vi "MFLI_Merge_Cluster.vi"(3 "MFL_Monitor Control":T1 {"Osc 3 Freq" min=0.0 max=510000.0 format="%#_11g"; "Osc 2 Freq" min=0.0 max=510000.0 format="%#_11g"; "Osc 1 Freq" min=0.0 max=510000.0 format="%#_11g"; "Osc 0 Freq" min=0.0 max=510000.0 format="%#_11g"}, 5 "MFL_Monitor Status":T2 {"Demod Sample out 3"."Aux In 1 (V)" format="%#_5p"; "Demod Sample out 3"."Aux In 0 (V)" format="%#_5p"; "Demod Sample out 3"."X (Vrms)" format="%#_5p"; "Demod Sample out 3"."Y (Vrms)" format="%#_5p"; "Demod Sample out 3"."Osc Phase (rad)" format="%#.3g"; "Demod Sample out 2"."Aux In 1 (V)" format="%#_5p"; "Demod Sample out 2"."Aux In 0 (V)" format="%#_5p"; "Demod Sample out 2"."X (Vrms)" format="%#_5p"; "Demod Sample out 2"."Y (Vrms)" format="%#_5p"; "Demod Sample out 2"."Osc Phase (rad)" format="%#.3g"; "Demod Sample out 1"."Aux In 1 (V)" format="%#_5p"; "Demod Sample out 1"."Aux In 0 (V)" format="%#_5p"; "Demod Sample out 1"."X (Vrms)" format="%#_5p"; "Demod Sample out 1"."Y (Vrms)" format="%#_5p"; "Demod Sample out 1"."Osc Phase (rad)" format="%#.3g"; "Demod Sample out 0"."Aux In 1 (V)" format="%#_5p"; "Demod Sample out 0"."Aux In 0 (V)" format="%#_5p"; "Demod Sample out 0"."X (Vrms)" format="%#_5p"; "Demod Sample out 0"."Y (Vrms)" format="%#_5p"; "Demod Sample out 0"."Osc Phase (rad)" format="%#.3g"}) -> (1 "MFL_Monitor":T4 {"Osc 3 Freq" min=0.0 max=510000.0 format="%#_11g"; "Osc 2 Freq" min=0.0 max=510000.0 format="%#_11g"; "Osc 1 Freq" min=0.0 max=510000.0 format="%#_11g"; "Osc 0 Freq" min=0.0 max=510000.0 format="%#_11g"; "Demod Sample out 3"."Aux In 1 (V)" format="%#_5p"; "Demod Sample out 3"."Aux In 0 (V)" format="%#_5p"; "Demod Sample out 3"."X (Vrms)" format="%#_5p"; "Demod Sample out 3"."Y (Vrms)" format="%#_5p"; "Demod Sample out 3"."Osc Phase (rad)" format="%#.3g"; "Demod Sample out 2"."Aux In 1 (V)" format="%#_5p"; "Demod Sample out 2"."Aux In 0 (V)" format="%#_5p"; "Demod Sample out 2"."X (Vrms)" format="%#_5p"; "Demod Sample out 2"."Y (Vrms)" format="%#_5p"; "Demod Sample out 2"."Osc Phase (rad)" format="%#.3g"; "Demod Sample out 1"."Aux In 1 (V)" format="%#_5p"; "Demod Sample out 1"."Aux In 0 (V)" format="%#_5p"; "Demod Sample out 1"."X (Vrms)" format="%#_5p"; "Demod Sample out 1"."Y (Vrms)" format="%#_5p"; "Demod Sample out 1"."Osc Phase (rad)" format="%#.3g"; "Demod Sample out 0"."Aux In 1 (V)" format="%#_5p"; "Demod Sample out 0"."Aux In 0 (V)" format="%#_5p"; "Demod Sample out 0"."X (Vrms)" format="%#_5p"; "Demod Sample out 0"."Y (Vrms)" format="%#_5p"; "Demod Sample out 0"."Osc Phase (rad)" format="%#.3g"})   [LabVIEW 2019]
uses:
  zurich_lock_in/MFLIMonitor_Cluster.ctl
  Equipment/Zurich Instruments LabOne/Public/Data/ziTypeDemodSampleEx.ctl
  zurich_lock_in/MFLIMonitor_Status_Cluster.ctl
  zurich_lock_in/MFLIMonitor_Control_Cluster.ctl
  Equipment/Zurich Instruments LabOne/Zurich Instruments LabOne.lvlib
panel:
  # "Oscillators"
  # "Output Amplitudes"
  # "Frequency (Hz)"
  # "Ampl (Vpk)"
  # "0"
  # "0"
  # "1"
  # "1"
  # "2"
  # "2"
  # "3"
  # "3"
  # "Oscillators"
  # "Output Amplitudes"
  # "Frequency (Hz)"
  # "Ampl (Vpk)"
  # "0"
  # "0"
  # "1"
  # "1"
  # "2"
  # "2"
  # "3"
  # "3"
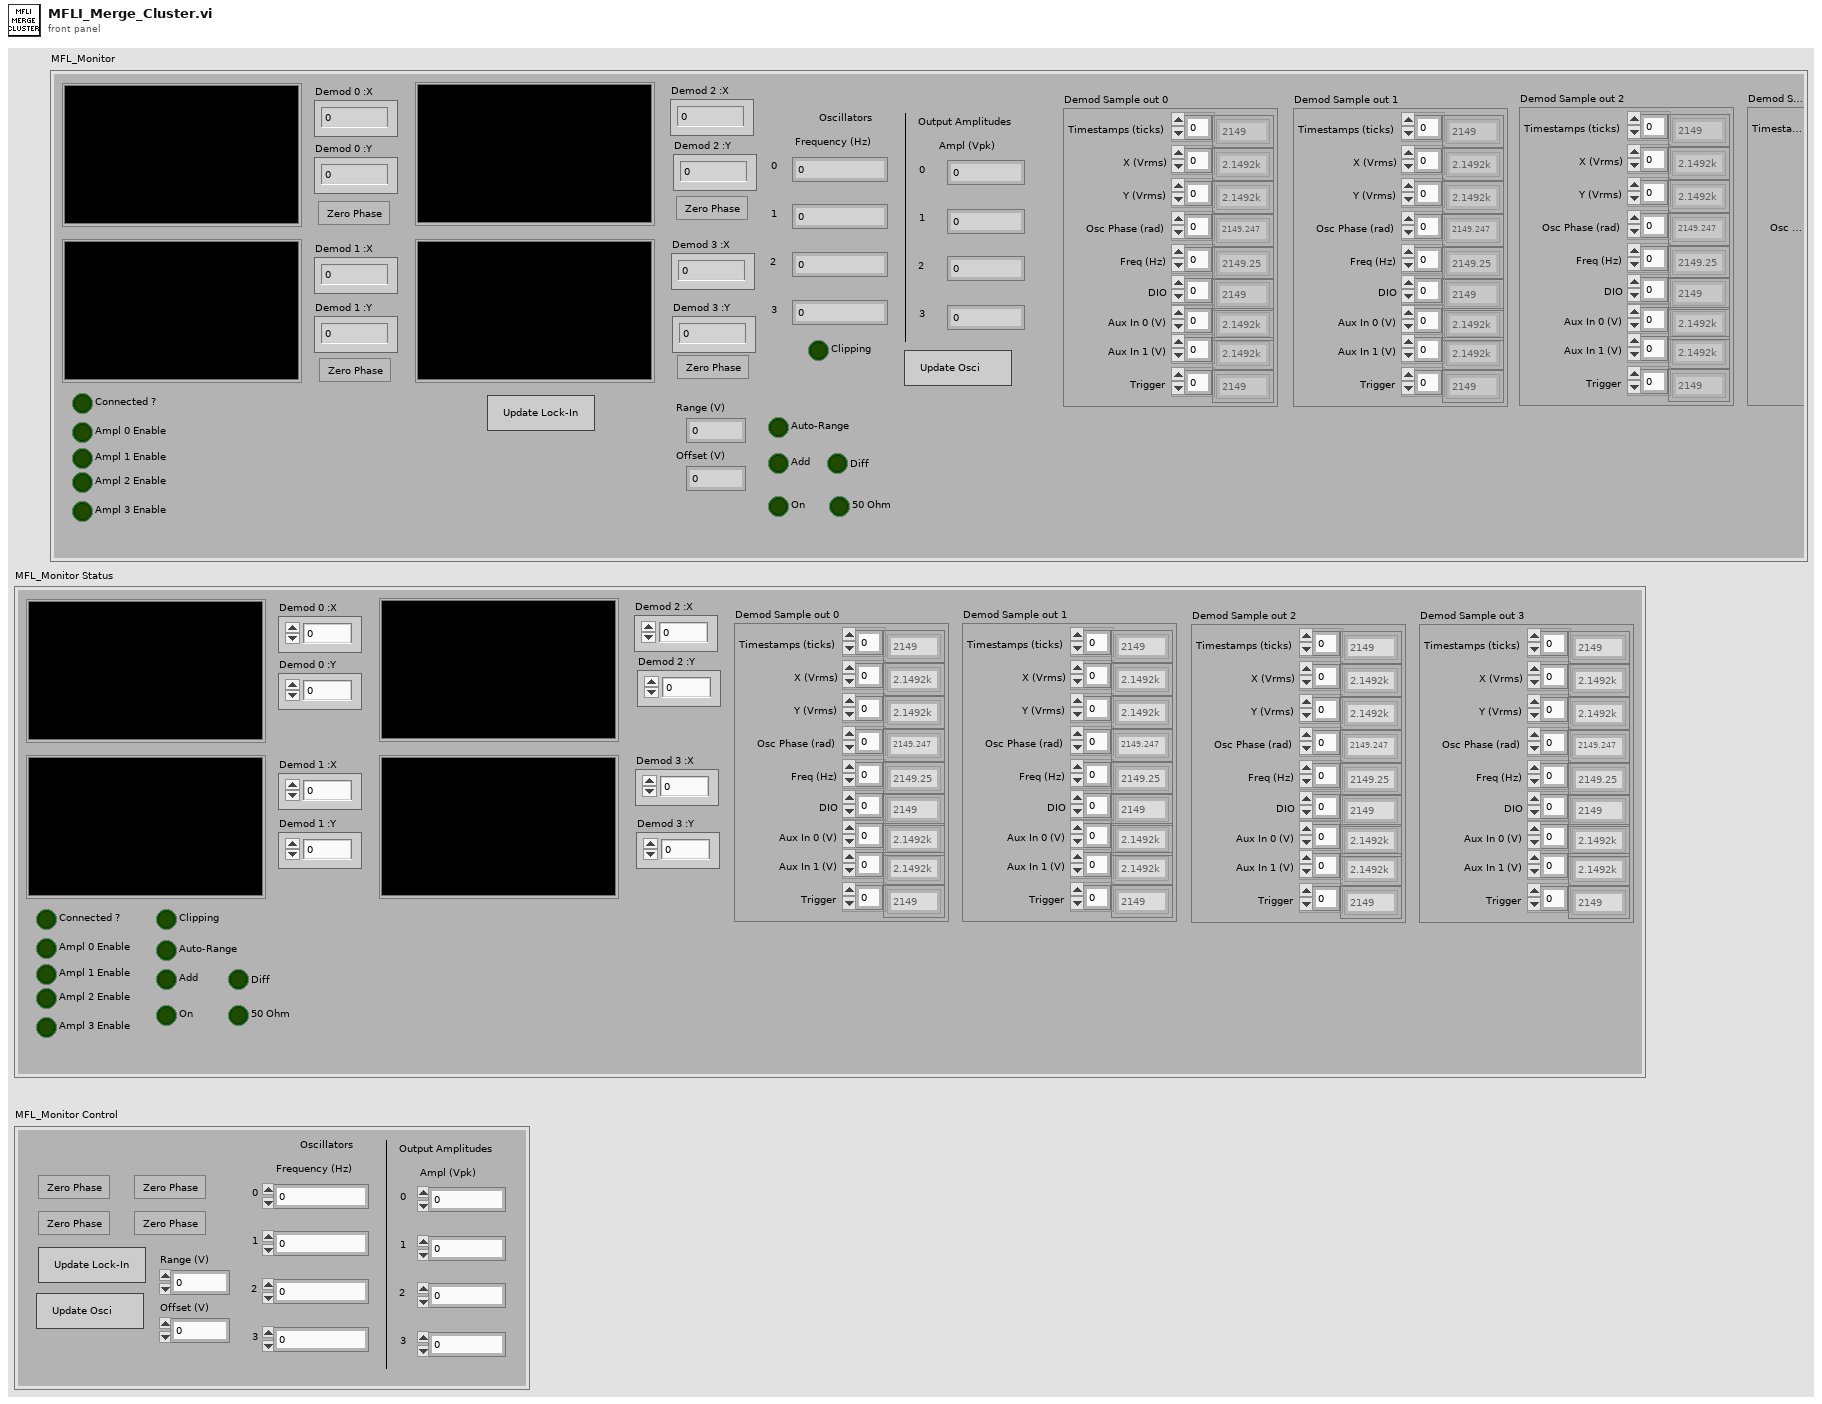
[diagram p1: front panel]
types:
  T1 = typedef "MFLIMonitor_Control_Cluster.ctl" = cluster{"Update Lock-In":bool, "Demod 0 Zero Phase":bool, "Demod 1 Zero Phase":bool, "Demod 2 Zero Phase":bool, "Demod 3 Zero Phase":bool, "Osc 0 Freq":dbl, "Osc 1 Freq":dbl, "Osc 2 Freq":dbl, "Osc 3 Freq":dbl, "Range (V)":dbl, "Offset (V)":dbl, "Ampl 0":dbl, "Ampl 1":dbl, "Ampl 2":dbl, "Ampl 3":dbl, "Update Osci":bool}
  T2 = typedef "MFLIMonitor_Status_Cluster.ctl" = cluster{"Demod 0":dbl[][], " Demod 1":dbl[][], "Demod 0 :X":dbl, "Demod 0 :Y ":dbl, "Demod 1 :X":dbl, "Demod 1 :Y ":dbl, " Demod 2":dbl[][], "Demod 3":dbl[][], "Demod 2 :X":dbl, "Demod 2 :Y ":dbl, "Demod 3 :X ":dbl, "Demod 3 :Y ":dbl, "Demod Sample out 0 ":T3, "Demod Sample out 1":T3, "Demod Sample out 2":T3, "Demod Sample out 3":T3, "Connected ?":bool, "Clipping":bool, "Auto-Range":bool, "Add":bool, "Diff":bool, "On":bool, "50 Ohm":bool, "Ampl 0 Enable":bool, "Ampl 1 Enable":bool, "Ampl 2 Enable":bool, "Ampl 3 Enable":bool}
  T3 = typedef "Zurich Instruments LabOne.lvlib/ziTypeDemodSampleEx.ctl" = cluster{"Timestamps (ticks)":u64[], "X (Vrms)":dbl[], "Y (Vrms)":dbl[], "Osc Phase (rad)":dbl[], "Freq (Hz)":dbl[], "DIO":u32[], "Aux In 0 (V)":dbl[], "Aux In 1 (V)":dbl[], "Trigger":u32[]}
  T4 = typedef "MFLIMonitor_Cluster.ctl" = cluster{"Demod 0":dbl[][], " Demod 1":dbl[][], "Demod 0 :X":dbl, "Demod 0 :Y ":dbl, "Demod 1 :X":dbl, "Demod 1 :Y ":dbl, " Demod 2":dbl[][], "Demod 3":dbl[][], "Demod 2 :X":dbl, "Demod 2 :Y ":dbl, "Demod 3 :X ":dbl, "Demod 3 :Y ":dbl, "Demod Sample out 0 ":T3, "Demod Sample out 1":T3, "Demod Sample out 2":T3, "Demod Sample out 3":T3, "Update Lock-In":bool, "Connected ?":bool, "Demod 0 Zero Phase":bool, "Demod 1 Zero Phase":bool, "Demod 2 Zero Phase":bool, "Demod 3 Zero Phase":bool, "Osc 0 Freq":dbl, "Osc 1 Freq":dbl, "Osc 2 Freq":dbl, "Osc 3 Freq":dbl, "Clipping":bool, "Range (V)":dbl, "Offset (V)":dbl, "Auto-Range":bool, "Add":bool, "Diff":bool, "On":bool, "50 Ohm":bool, "Ampl 0 Enable":bool, "Ampl 1 Enable":bool, "Ampl 2 Enable":bool, "Ampl 3 Enable":bool, "Ampl 0":dbl, "Ampl 1":dbl, "Ampl 2":dbl, "Ampl 3":dbl, "Update Osci":bool}
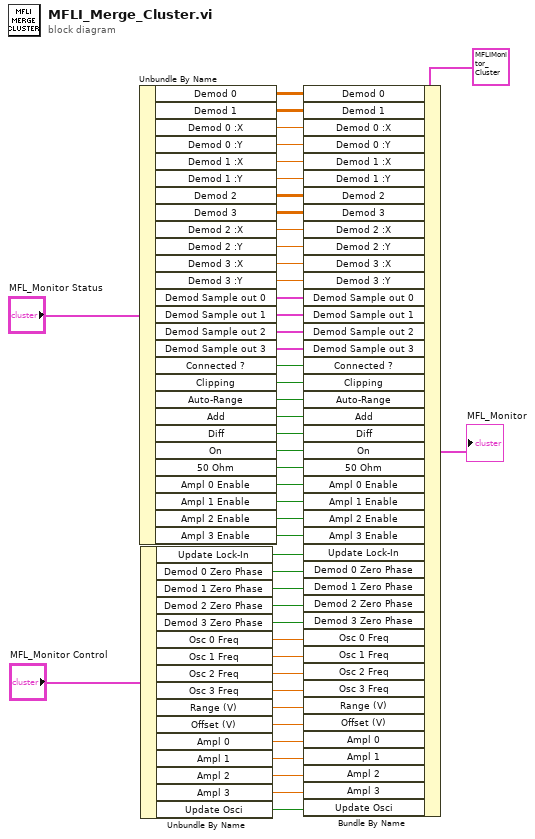
[diagram p0: block diagram]
diagram:
  n1 = Unbundle By Name("MFL_Monitor Status") -> ("Demod 0"=w44:dbl[][], "Demod 1"=w43:dbl[][], "Demod 0 :X"=w42:dbl, "Demod 0 :Y"=w41:dbl, "Demod 1 :X"=w40:dbl, "Demod 1 :Y"=w39:dbl, "Demod 2"=w38:dbl[][], "Demod 3"=w37:dbl[][], "Demod 2 :X"=w36:dbl, "Demod 2 :Y"=w35:dbl, "Demod 3 :X"=w34:dbl, "Demod 3 :Y"=w33:dbl, "Demod Sample out 0"=w32:T3, "Demod Sample out 1"=w31:T3, "Demod Sample out 2"=w30:T3, "Demod Sample out 3"=w29:T3, "Connected ?"=w28:bool, "Clipping"=w27:bool, "Auto-Range"=w26:bool, "Add"=w25:bool, "Diff"=w24:bool, "On"=w23:bool, "50 Ohm"=w22:bool, "Ampl 0 Enable"=w21:bool, "Ampl 1 Enable"=w20:bool, "Ampl 2 Enable"=w19:bool, "Ampl 3 Enable"=w18:bool)
  n2 = Unbundle By Name("MFL_Monitor Control") -> ("Update Lock-In"=w16:bool, "Demod 0 Zero Phase"=w15:bool, "Demod 1 Zero Phase"=w14:bool, "Demod 2 Zero Phase"=w13:bool, "Demod 3 Zero Phase"=w12:bool, "Osc 0 Freq"=w11:dbl, "Osc 1 Freq"=w10:dbl, "Osc 2 Freq"=w9:dbl, "Osc 3 Freq"=w8:dbl, "Range (V)"=w7:dbl, "Offset (V)"=w6:dbl, "Ampl 0"=w5:dbl, "Ampl 1"=w4:dbl, "Ampl 2"=w3:dbl, "Ampl 3"=w2:dbl, "Update Osci"=w1:bool)
  n3 = Bundle By Name(cluster=T4 {"Demod 0"=[], " Demod 1"=[], "Demod 0 :X"=0.0, "Demod 0 :Y "=0.0, "Demod 1 :X"=0.0, "Demod 1 :Y "=0.0, " Demod 2"=[], "Demod 3"=[], "Demod 2 :X"=0.0, "Demod 2 :Y "=0.0, "Demod 3 :X "=0.0, "Demod 3 :Y "=0.0, "Demod Sample out 0 "={"Timestamps (ticks)"=[], "X (Vrms)"=[], "Y (Vrms)"=[], "Osc Phase (rad)"=[], "Freq (Hz)"=[], "DIO"=[], "Aux In 0 (V)"=[], "Aux In 1 (V)"=[], "Trigger"=[]}, "Demod Sample out 1"={"Timestamps (ticks)"=[], "X (Vrms)"=[], "Y (Vrms)"=[], "Osc Phase (rad)"=[], "Freq (Hz)"=[], "DIO"=[], "Aux In 0 (V)"=[], "Aux In 1 (V)"=[], "Trigger"=[]}, "Demod Sample out 2"={"Timestamps (ticks)"=[], "X (Vrms)"=[], "Y (Vrms)"=[], "Osc Phase (rad)"=[], "Freq (Hz)"=[], "DIO"=[], "Aux In 0 (V)"=[], "Aux In 1 (V)"=[], "Trigger"=[]}, "Demod Sample out 3"={"Timestamps (ticks)"=[], "X (Vrms)"=[], "Y (Vrms)"=[], "Osc Phase (rad)"=[], "Freq (Hz)"=[], "DIO"=[], "Aux In 0 (V)"=[], "Aux In 1 (V)"=[], "Trigger"=[]}, "Update Lock-In"=FALSE, "Connected ?"=FALSE, "Demod 0 Zero Phase"=FALSE, "Demod 1 Zero Phase"=FALSE, "Demod 2 Zero Phase"=FALSE, "Demod 3 Zero Phase"=FALSE, "Osc 0 Freq"=0.0, "Osc 1 Freq"=0.0, "Osc 2 Freq"=0.0, "Osc 3 Freq"=0.0, "Clipping"=FALSE, "Range (V)"=0.0, "Offset (V)"=0.0, "Auto-Range"=FALSE, "Add"=FALSE, "Diff"=FALSE, "On"=FALSE, "50 Ohm"=FALSE, "Ampl 0 Enable"=FALSE, "Ampl 1 Enable"=FALSE, "Ampl 2 Enable"=FALSE, "Ampl 3 Enable"=FALSE, "Ampl 0"=0.0, "Ampl 1"=0.0, "Ampl 2"=0.0, "Ampl 3"=0.0, "Update Osci"=FALSE} ("MFL_Monitor"), "Demod 0"=w44, "Demod 1"=w43, "Demod 0 :X"=w42, "Demod 0 :Y"=w41, "Demod 1 :X"=w40, "Demod 1 :Y"=w39, "Demod 2"=w38, "Demod 3"=w37, "Demod 2 :X"=w36, "Demod 2 :Y"=w35, "Demod 3 :X"=w34, "Demod 3 :Y"=w33, "Demod Sample out 0"=w32, "Demod Sample out 1"=w31, "Demod Sample out 2"=w30, "Demod Sample out 3"=w29, "Connected ?"=w28, "Clipping"=w27, "Auto-Range"=w26, "Add"=w25, "Diff"=w24, "On"=w23, "50 Ohm"=w22, "Ampl 0 Enable"=w21, "Ampl 1 Enable"=w20, "Ampl 2 Enable"=w19, "Ampl 3 Enable"=w18, "Update Lock-In"=w16, "Demod 0 Zero Phase"=w15, "Demod 1 Zero Phase"=w14, "Demod 2 Zero Phase"=w13, "Demod 3 Zero Phase"=w12, "Osc 0 Freq"=w11, "Osc 1 Freq"=w10, "Osc 2 Freq"=w9, "Osc 3 Freq"=w8, "Range (V)"=w7, "Offset (V)"=w6, "Ampl 0"=w5, "Ampl 1"=w4, "Ampl 2"=w3, "Ampl 3"=w2, "Update Osci"=w1) -> (→"MFL_Monitor":T4)
